vi "SubPanel_Path.vi"() -> (3 "SubPanelPath":path)   [LabVIEW 2014, in "SubPanelModule.lvlib"]
uses:
  SubPanelModule.lvlib
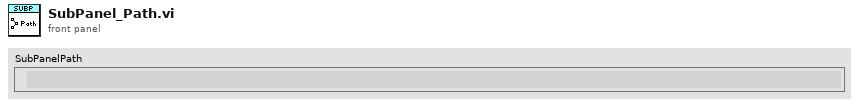
[diagram p1: front panel]
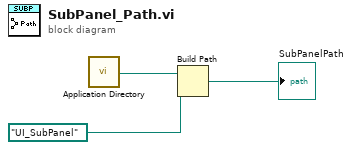
[diagram p0: block diagram]
diagram:
  n1 = call <vilib>:"Application Directory.vi"() -> ("Application Directory"=w1:path)
  n2 = Build Path(base path=w1, name or relative path=path "UI_SubPanel") -> (appended path=→"SubPanelPath":path)
